vi "test_libssh2_channel_wait_eof.vi"() -> ()   [LabVIEW 2017, in "integration_tests.lvlib"]
uses:
  integration_tests.lvlib
  libssh2/libssh2_channel_open_ex.vi
  libssh2/libssh2_channel_process_startup.vi
  support/support.lvlib
  libssh2/libssh2.lvlib
  <vilib>/PNR/Transparent Assertions/Transparent Assertions/Transparent Assertions.lvlib
panel:
  out "error out":errorcluster
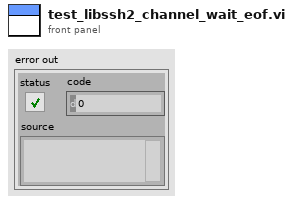
[diagram p1: front panel]
types:
  T1 = typedef "libssh2.lvlib/Session Refnum.ctl" = refnum<k1>
  T2 = typedef "libssh2.lvlib/Channel Refnum.ctl" = refnum<k1>
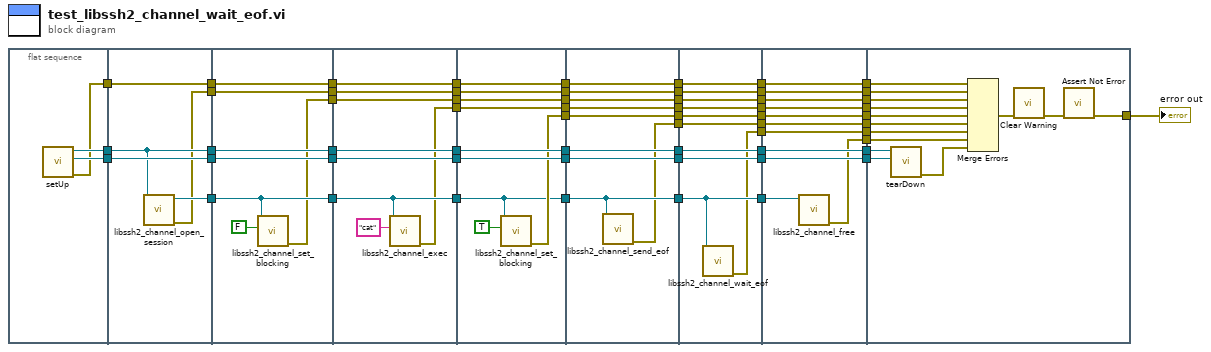
[diagram p0: block diagram]
diagram:
  n1 = flat-sequence {
    tunnel: [w62] -> w59
    tunnel: [w61] -> w58
    tunnel: [w60] -> w57
    tunnel: w59 -> [w66]
    tunnel: w58 -> [w67]
    tunnel: [w66] -> w34
    tunnel: [w67] -> w32
    tunnel: [w65] -> w26
    tunnel: w57 -> [w64]
    tunnel: [w64] -> w30
    tunnel: [w63] -> w28
    tunnel: w34 -> [w74]
    tunnel: [w74] -> w33
    tunnel: w32 -> [w73]
    tunnel: [w73] -> w31
    tunnel: w30 -> [w72]
    tunnel: [w72] -> w29
    tunnel: w28 -> [w71]
    tunnel: [w71] -> w27
    tunnel: w26 -> [w70]
    tunnel: [w70] -> w25
    tunnel: [w68] -> w24
    tunnel: w33 -> [w82]
    tunnel: [w82] -> w20
    tunnel: w31 -> [w81]
    tunnel: [w81] -> w18
    tunnel: w29 -> [w80]
    tunnel: [w80] -> w16
    tunnel: w27 -> [w79]
    tunnel: [w79] -> w14
    tunnel: w25 -> [w78]
    tunnel: [w78] -> w12
    tunnel: [w76] -> w10
    tunnel: w24 -> [w75]
    tunnel: [w75] -> w8
    tunnel: w20 -> [w91]
    tunnel: [w91] -> w19
    tunnel: w18 -> [w90]
    tunnel: [w90] -> w17
    tunnel: w16 -> [w89]
    tunnel: [w89] -> w15
    tunnel: w14 -> [w88]
    tunnel: [w88] -> w13
    tunnel: w12 -> [w83]
    tunnel: [w83] -> w11
    tunnel: w10 -> [w87]
    tunnel: [w87] -> w9
    tunnel: w8 -> [w86]
    tunnel: [w86] -> w7
    tunnel: [w84] -> w6
    tunnel: w19 -> [w100]
    tunnel: [w100] -> w50
    tunnel: w17 -> [w99]
    tunnel: [w99] -> w48
    tunnel: w15 -> [w98]
    tunnel: [w98] -> w46
    tunnel: w13 -> [w97]
    tunnel: [w97] -> w44
    tunnel: w11 -> [w96]
    tunnel: [w96] -> w42
    tunnel: [w95] -> w40
    tunnel: w9 -> [w94]
    tunnel: [w94] -> w37
    tunnel: w7 -> [w93]
    tunnel: [w93] -> w23
    tunnel: w6 -> [w92]
    tunnel: [w92] -> w5
    tunnel: w50 -> [w110]
    tunnel: [w110] -> w49
    tunnel: w48 -> [w109]
    tunnel: [w109] -> w47
    tunnel: w46 -> [w108]
    tunnel: [w108] -> w45
    tunnel: w44 -> [w107]
    tunnel: [w107] -> w43
    tunnel: w42 -> [w105]
    tunnel: [w105] -> w41
    tunnel: w40 -> [w106]
    tunnel: [w106] -> w39
    tunnel: w37 -> [w104]
    tunnel: [w104] -> w36
    tunnel: w23 -> [w103]
    tunnel: [w103] -> w22
    tunnel: w5 -> [w102]
    tunnel: [w102] -> w4
    tunnel: [w101] -> w2
    tunnel: w49 -> [w121]
    tunnel: w47 -> [w120]
    tunnel: [w121] -> w56
    tunnel: [w120] -> w55
    tunnel: [w119] -> w54
    tunnel: w45 -> [w118]
    tunnel: [w118] -> w53
    tunnel: w43 -> [w117]
    tunnel: [w117] -> w52
    tunnel: w41 -> [w116]
    tunnel: w39 -> [w115]
    tunnel: [w115] -> w38
    tunnel: w36 -> [w114]
    tunnel: [w114] -> w35
    tunnel: w22 -> [w113]
    tunnel: [w113] -> w21
    tunnel: w4 -> [w112]
    tunnel: [w112] -> w3
    tunnel: w2 -> [w111]
    tunnel: [w111] -> w1
    tunnel: w56 -> [w135]
    tunnel: w55 -> [w134]
    tunnel: [w133] -> w51
    tunnel: w54 -> [w131]
    tunnel: w53 -> [w130]
    tunnel: w52 -> [w128]
    tunnel: w38 -> [w127]
    tunnel: w35 -> [w126]
    tunnel: w21 -> [w125]
    tunnel: w3 -> [w124]
    tunnel: w1 -> [w123]
    frame #0 {
      n2 = call "setUp.vi"() -> ("error out"=w60:errorcluster, "connection ID"=w61:refnum<k5>, "session"=w62:T1)  [unwired: 9 in]
    }
    frame #1 {
      n3 = call "libssh2_channel_open_session.vi"("session"=w66) -> ("error out"=w63:errorcluster, "channel"=w65:T2)  [unwired: 9 in]
    }
    frame #2 {
      n4 = call "libssh2_channel_set_blocking.vi"("blocking"=FALSE, "channel"=w70) -> ("error out"=w68:errorcluster)  [unwired: 9 in]
    }
    frame #3 {
      n5 = call "libssh2_channel_exec.vi"("command"="cat", "channel"=w78) -> ("error out"=w76:errorcluster)  [unwired: 9 in]
    }
    frame #4 {
      n6 = call "libssh2_channel_set_blocking.vi"("blocking"=TRUE, "channel"=w83) -> ("error out"=w84:errorcluster)  [unwired: 9 in]
    }
    frame #5 {
      n7 = call "libssh2_channel_send_eof.vi"("channel"=w96) -> ("error out"=w95:errorcluster)  [unwired: 10 in]
    }
    frame #6 {
      n8 = call "libssh2_channel_wait_eof.vi"("channel"=w105) -> ("error out"=w101:errorcluster)  [unwired: 10 in]
    }
    frame #7 {
      n9 = call "libssh2_channel_free.vi"("channel"=w116) -> ("error out"=w119:errorcluster)  [unwired: 10 in]
    }
    frame #8 {
      n10 = call "tearDown.vi"("connection ID"=w134, "session"=w135) -> ("error out"=w132:errorcluster)  [unwired: 9 in]
      n11 = Merge Errors(w130, w128, w125, w126, w124, w127, w123, w131, w132) -> (w129:errorcluster)
      n12 = call "Clear Warning.vi"("error in (no error)"=w129) -> ("error out"=w122:errorcluster)  [unwired: 10 in]
      n13 = call <vilib>:"Assert Not Error.vi"("error in (no error)"=w122) -> ("error out"=w133:errorcluster)  [unwired: 10 in]
    }
  }
  "error out" <- w51
